vi "Constructor.vi"(8 "error in":errorcluster, 9 "Value":bool, 10 "Name":string, 11 "Boolean in":refnum<class "Boolean.lvclass">) -> (0 "error out":errorcluster, 3 "Boolean out":refnum<class "Boolean.lvclass">)   [LabVIEW 2021, in "ProligentXMLGenerator.lvlib" / "Boolean.lvclass"]
uses:
  Boolean.lvclass
  Boolean.lvclass/Boolean.ctl
  Attribute/Attribute.lvclass
  C:/Projects/proligent-xml-generator-labview/src/ProligentXMLGenerator/Base/Attribute/Attribute.lvclass
  C:/Projects/proligent-xml-generator-labview/src/ProligentXMLGenerator/Base/Boolean/Boolean.lvclass
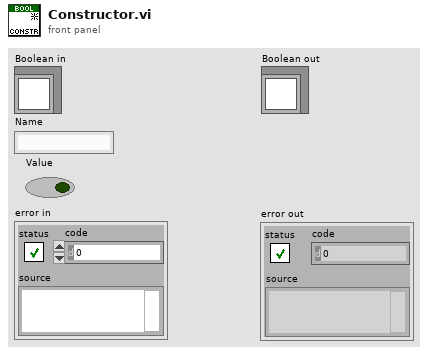
[diagram p1: front panel]
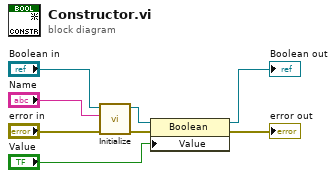
[diagram p0: block diagram]
diagram:
  n1 = call "Initialize.vi"("error in"="error in", "Name"="Name", "Attribute in"="Boolean in") -> ("error out"=w4:errorcluster, "Attribute out"=w3:refnum<class "Boolean.lvclass">)  [unwired: 7 in]
  n2 = property on="Property Node" class="Boolean"(reference=w3, error in=w4, "Value"="Value") -> (reference out=→"Boolean out":refnum<class "Boolean.lvclass">, error out=→"error out":errorcluster)
